vi "construct_response_instr_status.vi"(0 "command in":T9=enum."get_instrument_status", 1 "Status":T8, 5 "generic_info":string, 9 "Config":T1, 11 "error in (no error) 2":errorcluster, 12 "source":string) -> (6 "Multipart message":string[](array[string]), 14 "parameters JSON":string, 15 "error out 2":errorcluster)   [LabVIEW 2019, in "mmW_commands.lvlib"]
uses:
  mmW_commands.lvlib
  TypeDefs/commands.ctl
  TypeDefs/response status.ctl
  mmw_instrument/src_LabVIEW/Host/SubVIs/Shared/Config state.ctl
  mmw_instrument/src_LabVIEW/Host/SubVIs/mmWave instrument_class/System info.ctl
  mmw_instrument/src_LabVIEW/Host/SubVIs/mmWave instrument_class/System state.ctl
  mmw_instrument/src_LabVIEW/Host/SubVIs/mmWave instrument_class/Instrument state.ctl
  mmw_instrument/src_LabVIEW/Host/SubVIs/mmWave instrument_class/Instrument mode.ctl
  mmw_instrument/src_LabVIEW/Host/SubVIs/mmWave instrument_class/Sync mode.ctl
  mmw_instrument/src_LabVIEW/Host/SubVIs/mmWave instrument_class/RF port info.ctl
  typedefs/Response_paramaters.ctl
  typedefs/datatypes_.ctl
  <vilib>/addons/_JKI.lib/Serialization/JSON/JKI JSON Serialization.lvlib
  mmw_instrument/src_LabVIEW/Host/SubVIs/mmWave instrument_class/mmWave instrument.lvclass
  mmw_instrument/src_LabVIEW/Host/SubVIs/Shared/Shared.lvlib
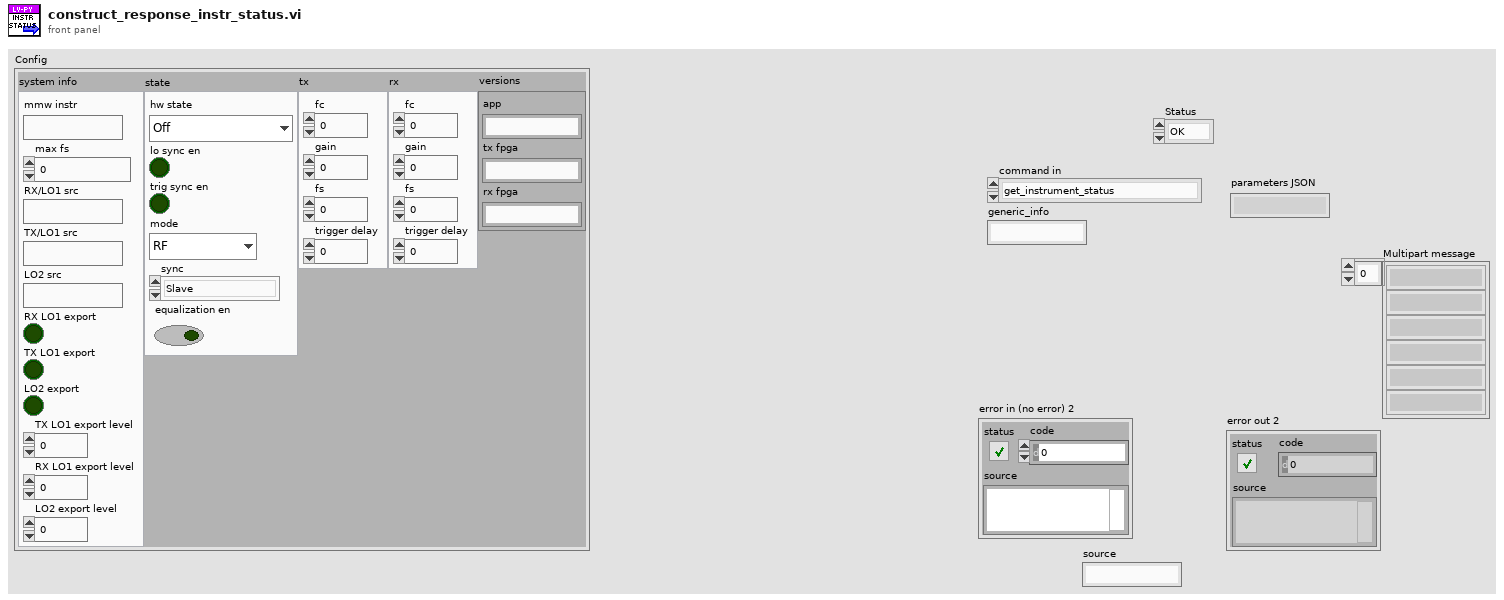
[diagram p1: front panel]
types:
  T1 = typedef "Shared.lvlib/Config state.ctl" = cluster{"system info":T2, "state":T3, "tx":T7, "rx":T7, "versions":cluster{"app":string, "tx fpga":string, "rx fpga":string}}
  T2 = typedef "mmWave instrument.lvclass/System info.ctl" = cluster{"mmw instr":string, "max fs":dbl, "RX/LO1 src":string, "TX/LO1 src":string, "LO2 src":string, "RX LO1 export":bool, "TX LO1 export":bool, "LO2 export":bool, "TX LO1 export level":dbl, "RX LO1 export level":dbl, "LO2 export level":dbl}
  T3 = typedef "mmWave instrument.lvclass/System state.ctl" = cluster{"hw state":T4, "lo sync en":bool, "trig sync en":bool, "mode":T5, "sync":T6, "equalization en":bool}
  T4 = typedef "mmWave instrument.lvclass/Instrument state.ctl" = enum16{"Off", "Initialization", "Configuration", "Running", "Calibration"}
  T5 = typedef "mmWave instrument.lvclass/Instrument mode.ctl" = enum16{"RF", "IF", "BB"}
  T6 = typedef "mmWave instrument.lvclass/Sync mode.ctl" = enum16{"Slave", "Master"}
  T7 = typedef "mmWave instrument.lvclass/RF port info.ctl" = cluster{"fc":dbl, "gain":dbl, "fs":dbl, "trigger delay":dbl}
  T8 = typedef "mmW_commands.lvlib/response status.ctl" = enum16{"OK", "Error", "Warning", "Unknown"}
  T9 = typedef "mmW_commands.lvlib/commands.ctl" = enum16{"configure_fs", "configure_rf", "configure_trigger", "equalization_enable", "equalization_start", "lo_sync_enable", "equalization_stop", "get_instrument_status", "get_versions", "initialize_hw", "pop_rx", "set_log_level", "Shutdown", "start", "start_instrument_app", "stop", "trans", "transceive", "trigger_burst", "trigger_sync_enable", "Write TX", "resp_generic", "resp_waveform", "send_trigger", "fetch", "transceive2"}
  T10 = typedef "mmW_commands.lvlib/datatypes_.ctl" = enum16{"none", "string", "interleaved_I16", "interleaved_I32", "I16_array", "I32_array", "JSONstring"}
  T11 = typedef "mmW_commands.lvlib/Response_paramaters.ctl" = cluster{"generic_info":string, "datatype":string, "source":string}
  T12 = enum16{"big-endian, network order", "native, host order", "little-endian"}
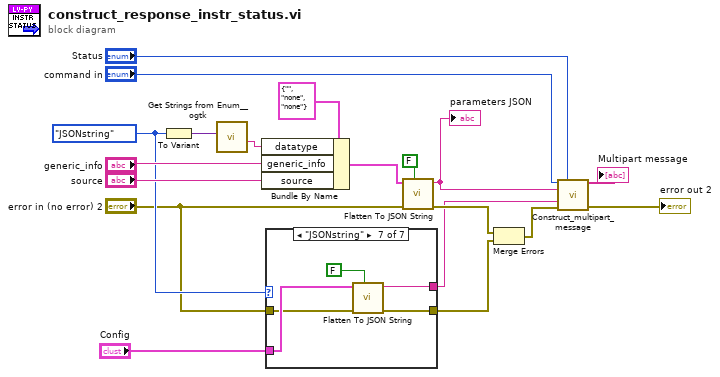
[diagram p0: block diagram]
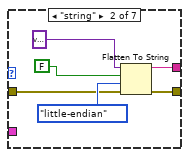
[diagram p3: hidden frame]
diagram:
  w3 = datatypes_."JSONstring" ("datatype")
  n1 = To Variant(anything=w3) -> (Variant=w10:variant)
  n2 = call <userlib>:"Get Strings from Enum__ogtk.vi"("Enum"=w10) -> ("String Value"=w9:string)  [unwired: 7 in, 3 out]
  n3 = Bundle By Name(cluster=T11 {"generic_info"="", "datatype"="none", "source"="none"} ("response data"), "datatype"=w9, "generic_info"="generic_info", "source"="source") -> (w18:T11)
  n4 = case shown="\"JSONstring\"" w3 {
    tunnel: [w20 w23 w27 w28 w29 w30 w33] -> w7
    tunnel: [_ w22 _ _ _ _ w32] -> w6
    tunnel: "error in (no error) 2" -> [w20 w21 w27 w28 w29 w30 w31]
    tunnel: "Config" -> [_ _ _ _ _ _ w34]
    frame "none", Default {
    }
    frame "string" {
      n5 = Flatten To String(anything=variant ("data in"), prepend array or string size? (T)=FALSE, byte order (0:big-endian, network order)=T12."little-endian", error in (no error)=w21) -> (data string=w22:string, error out=w23:errorcluster)  [unwired: 1 out]
    }
    frame "interleaved_I16" {
    }
    frame "interleaved_I32" {
    }
    frame "I16_array" {
    }
    frame "I32_array" {
    }
    frame "JSONstring" {
      n6 = call <vilib>:"Flatten To JSON String.vi"("Multiline (T)"=FALSE, "error in (no error)"=w31, "Variant"=w34) -> ("error out"=w33:errorcluster, "JSON String"=w32:string)  [unwired: 7 in]
    }
  }
  n7 = call <vilib>:"Flatten To JSON String.vi"("Multiline (T)"=FALSE, "error in (no error)"="error in (no error) 2", "Variant"=w18) -> ("error out"=w8:errorcluster, "JSON String"=w15:string)  [unwired: 7 in]
  "parameters JSON" <- w15
  n8 = Merge Errors(w8, w7) -> (w5:errorcluster)
  n9 = call "Construct_multipart_message.vi"("command"="command in", "Status"="Status", "parameters (JSON)"=w15, "data in"=w6, "error in (no error)"=w5) -> ("Multipart message"=→"Multipart message":string[], "error out"=→"error out 2":errorcluster)  [unwired: 7 in, 2 out]
